vi "testRSASign&VerifyInvalidKey.vi"(8 "error in (no error)":errorcluster, 11 "TestCase in":refnum<class "TestRSA.lvclass">) -> (0 "error out":errorcluster, 3 "TestCase out":refnum<class "TestRSA.lvclass">)   [LabVIEW 2021, in "TestRSA.lvclass"]
uses:
  TestRSA.lvclass
  Source Code/Asymmetric Encryption/RSA/HashingAlgorithm.ctl
  Source Code/Asymmetric Encryption/RSA/RSASignaturePadding.ctl
  <vilib>/addons/_JKI Toolkits/VI Tester/TestCase.llb/TestCase.lvclass
  Source Code/Asymmetric Encryption/dotNET Crypto Asymmetric Encryption.lvlib
  Source Code/Key Management/dotNET Crypto Key Management.lvlib
  Source Code/Utility/dotNET Crypto Utility.lvlib
  C:/Program Files (x86)/National Instruments/LabVIEW 2021/vi.lib/addons/_JKI Toolkits/VI Tester/TestCase.llb/TestCase.lvclass
panel:
  out "public key length":i32
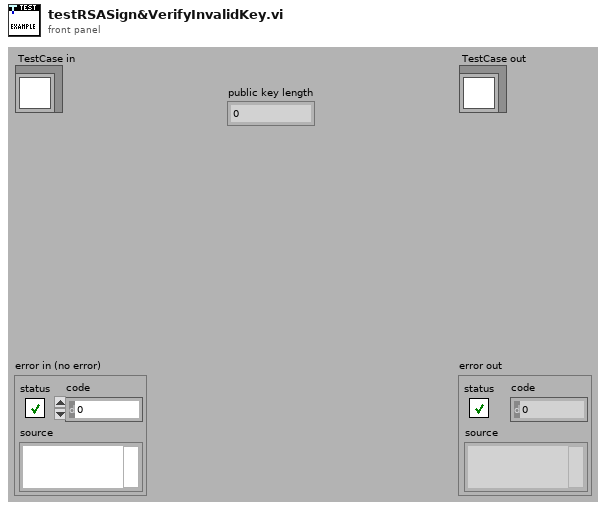
[diagram p1: front panel]
types:
  T1 = typedef "dotNET Crypto Asymmetric Encryption.lvlib/RSASignaturePadding.ctl" = enum16{"Pkcs1", "Pss"}
  T2 = typedef "dotNET Crypto Utility.lvlib/HashingAlgorithm.ctl" = enum16{"MD5", "SHA1", "SHA256", "SHA384", "SHA512"}
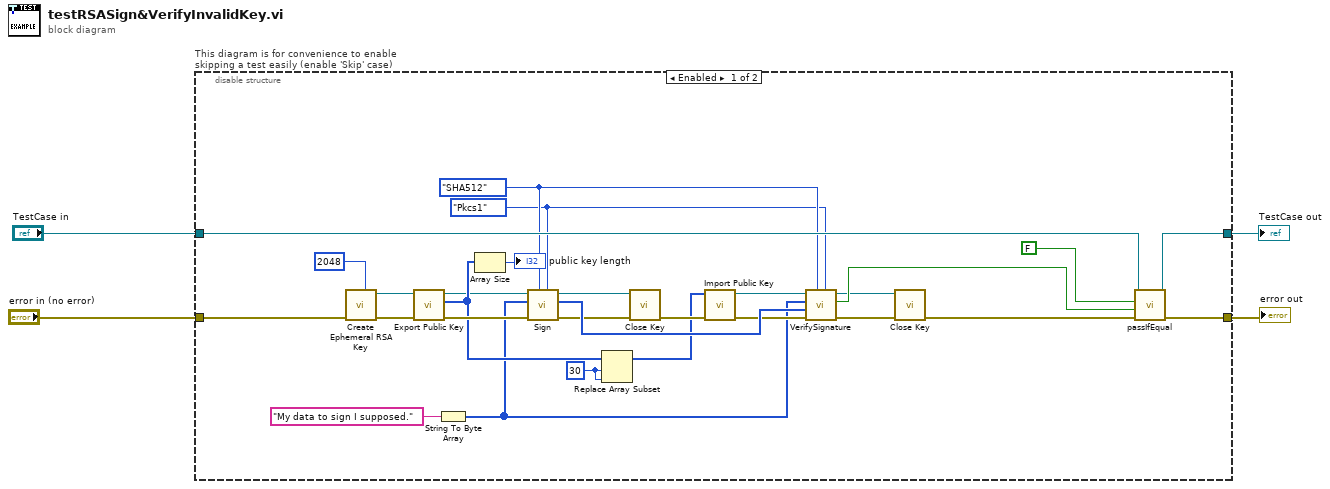
[diagram p0: block diagram]
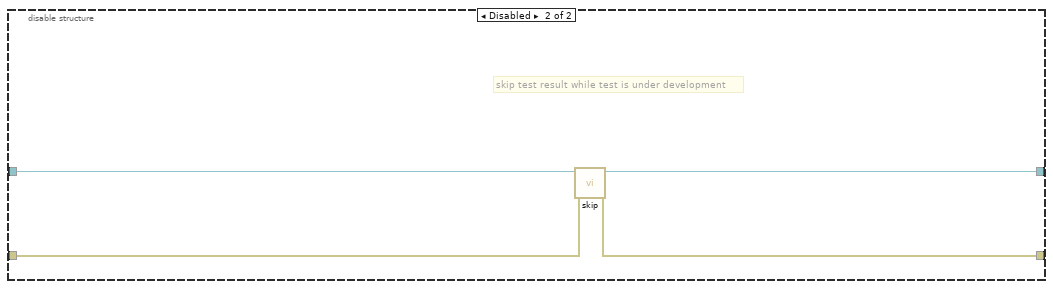
[diagram p2: hidden frame]
diagram:
  n1 = disable-structure "This diagram is for convenience to enable skipping a test easily (enable 'Skip' case)" shown="Enabled" {
    disable-tunnel: "TestCase in" -> [w32 w36]
    disable-tunnel: [w31 w34] -> w1
    disable-tunnel: [w30 w35] -> w3
    disable-tunnel: "error in (no error)" -> [w29 w33]
    frame Enabled {
      w23 = 30 ("index")
      w27 = RSASignaturePadding."Pkcs1" ("RSASignPadding")
      w28 = HashingAlgorithm."SHA512" ("HashingAlgorithm")
      n2 = call "Create Ephemeral RSA Key.vi"("Key Length (2048)"=2048 ("keySize (2048 bit)"), "error in (no error)"=w29) -> ("error out"=w15:errorcluster, "CngKey out"=w16:refnum<k24>)  [unwired: 8 in]
      n3 = call "Export Public Key.vi"("error in (no error)"=w15, "CngKey ref in"=w16) -> ("error out"=w14:errorcluster, "Public Key"=w13:u8[], "CngKey ref out"=w12:refnum<k24>)  [unwired: 7 in]
      n4 = String To Byte Array(string="My data to sign I supposed.") -> (unsigned byte array=w5:u8[])
      n5 = Array Size(array=w13) -> (size(s)=→"public key length":i32)
      n6 = call "Sign.vi"("RSASignPadding"=w27, "HashingAlgorithm"=w28, "error in (no error)"=w14, "Data in"=w5, "CngKey in"=w12) -> ("error out"=w10:errorcluster, "Signature out"=w18:u8[], "CngKey out"=w11:refnum<k24>)  [unwired: 4 in]
      n7 = Replace Array Subset(array=w13, new element=w23, index=w23) -> (w7:u8[])
      n8 = call "Close Key.vi"("error in (no error)"=w10, "CngKey in"=w11) -> ("error out"=w9:errorcluster)  [unwired: 9 in]
      n9 = call "Import Public Key.vi"("error in (no error)"=w9, "PublicKeyBlob"=w7) -> ("error out"=w8:errorcluster, "Imported CngKey out"=w6:refnum<k24>)  [unwired: 8 in]
      n10 = call "VerifySignature.vi"("RSASignPadding"=w27, "HashingAlgorithm"=w28, "error in (no error)"=w8, "Signature in"=w18, "Data in"=w5, "CngKey in"=w6) -> ("error out"=w26:errorcluster, "Verified?"=w21:bool, "CngKey out"=w19:refnum<k24>)  [unwired: 3 in]
      n11 = call "Close Key.vi"("error in (no error)"=w26, "CngKey in"=w19) -> ("error out"=w20:errorcluster)  [unwired: 9 in]
      n12 = call-dynamic "passIfEqual.vi"("error in (no error)"=w20, "y"=w21, "x"=FALSE, "TestCase in"=w32) -> ("error out"=w30:errorcluster, "TestCase out"=w31:refnum<class "TestRSA.lvclass">)  [unwired: 6 in]
    }
    frame Disabled {
      # "skip test result while test is under development"
      n13 = call <vilib>:"skip.vi"("error in (no error)"=w33, "TestCase in"=w36) -> ("error out"=w35:errorcluster, "TestCase out"=w34:refnum<class "TestRSA.lvclass">)  [unwired: 8 in]
    }
  }
  "error out" <- w3
  "TestCase out" <- w1
